vi "Eigenvalues.vi"(1 "Number of Rotations (100)":i32, 2 "n":i32, 3 "A":sgl[](array[numeric])) -> (0 "eigenvalues":sgl[](array[numeric]))   [LabVIEW 2020]
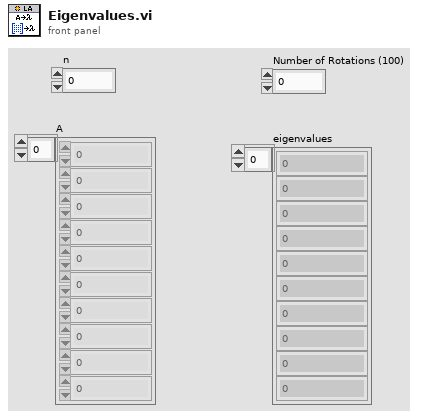
[diagram p1: front panel]
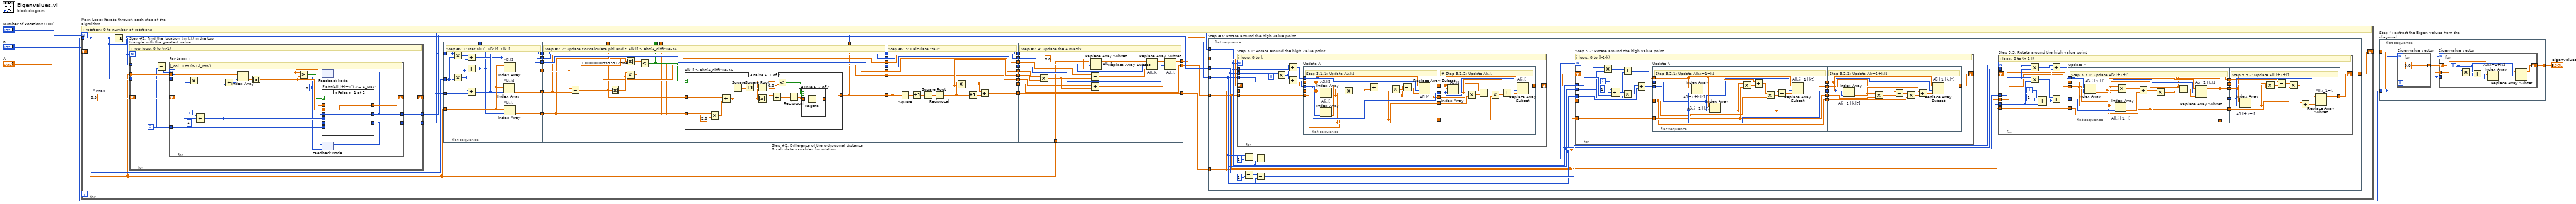
[diagram p0: block diagram]
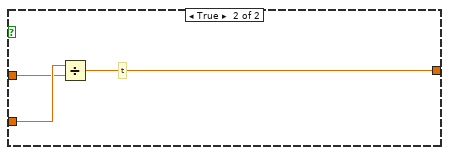
[diagram p3: hidden frame]
diagram:
  n1 = for "Main Loop: Iterate through each step of the algorithm" {
    N: "Number of Rotations (100)" -> [_]
    tunnel: "n" -> [w35]
    shift-right: [w6] -> w2
    shift-left: "A" -> [w25]
    w37 = sgl 0.0  # A max
    # "i_rotation: 0 to number_of_rotations"
    n2 = Decrement(x=w35) -> (x-1=w36:i32)
    n3 = for "Step #1: Find the location (in k,l) in the top triangle with the greatest value" {
      N: w36 -> [_]
      tunnel: w36 -> [w255]
      shift-right: [w259] -> _
      shift-left: w37 -> [w257]
      tunnel: [w258] -> w8
      tunnel: [w256] -> w7
      tunnel: w25 -> [w254]
      tunnel: w35 -> [w253]
      i -> [w252]
      # "i_row loop, 0 to (n-1)"
      n4 = Subtract(x=w255, y=w252) -> (x-y=w260:i32)
      n5 = for "For Loop: j" {
        N: w260 -> [_]
        shift-right: [w269] -> w259
        shift-left: w257 -> [w268]
        tunnel: [w261] -> w258
        tunnel: [w265] -> w256
        tunnel: w254 -> [w278]
        tunnel: w252 -> [w267]
        tunnel: w253 -> [w276]
        i -> [w272]
        w262 = 0
        # "j_col, 0 to (n-1-i_row)"
        n6 = Multiply(x=w276, y=w267) -> (x*y=w274:i32)
        n7 = Compound Arithmetic op=ADD(w272, w267, 1 ("value")) -> (w264:i32)
        n8 = Add(x=w274, y=w264) -> (x+y=w273:i32)
        n9 = Index Array(array=w278, index=w273) -> (element=w275:sgl)
        n10 = Absolute Value(x=w275) -> (abs(x)=w270:sgl)
        n11 = Greater Or Equal?(x=w270, y=w268) -> (x >= y?=w271:bool)
        n12 = feedback #1(w262) -> (w263:i32)
        n13 = feedback #2(w262) -> (w266:i32)
        n14 = case "if abs(A[i,j+i+1]) >= A_Max:" shown="False" w271 {
          tunnel: [w281 w284] -> w269
          tunnel: w270 -> [_ w284]
          tunnel: w268 -> [w281 _]
          tunnel: w267 -> [_ w283]
          tunnel: [w280 w283] -> w265
          tunnel: w266 -> [w280 _]
          tunnel: w264 -> [_ w282]
          tunnel: [w279 w282] -> w261
          tunnel: w263 -> [w279 _]
          frame False {
          }
          frame True {
          }
        }
        n15 = feedback-in #1(w261) -> ()
        n16 = feedback-in #2(w265) -> ()
      }
    }
    n17 = flat-sequence "Step #2: Difference of the orthogonal distance & calculate variables for rotation" {
      tunnel: [w45] -> w32
      tunnel: [w44] -> w31
      tunnel: [w43] -> w30
      tunnel: w7 -> [w49]
      tunnel: w35 -> [w48]
      tunnel: w8 -> [w47]
      tunnel: w25 -> [w46]
      tunnel: [w38] -> w21
      tunnel: [w40] -> w20
      tunnel: [w39] -> w17
      tunnel: [w38] -> _
      tunnel: [w53] -> w29
      tunnel: w32 -> [w55]
      tunnel: w31 -> [w54]
      tunnel: w30 -> [w50]
      tunnel: [w58] -> w22
      tunnel: w21 -> [w58]
      tunnel: w20 -> [w57]
      tunnel: [w57] -> w19
      tunnel: w17 -> [w56]
      tunnel: [w56] -> w16
      tunnel: [w50] -> w14
      tunnel: [w55] -> w12
      tunnel: [w54] -> w10
      tunnel: [w53] -> _
      tunnel: [w52] -> _
      tunnel: [w51] -> _
      tunnel: [w50] -> _
      tunnel: w29 -> [w91]
      tunnel: [w91] -> w28
      tunnel: [w90] -> w27
      tunnel: [w89] -> w26
      tunnel: [w88] -> w23
      tunnel: w22 -> [w88]
      tunnel: w19 -> [w87]
      tunnel: [w87] -> w18
      tunnel: w16 -> [w86]
      tunnel: [w86] -> w15
      tunnel: w14 -> [w85]
      tunnel: [w85] -> w13
      tunnel: w12 -> [w84]
      tunnel: [w84] -> w11
      tunnel: w10 -> [w83]
      tunnel: [w83] -> w9
      tunnel: [w112] -> w33
      tunnel: [w113] -> w34
      tunnel: w28 -> [w111]
      tunnel: w27 -> [w113]
      tunnel: w26 -> [w112]
      tunnel: w25 -> [w99]
      tunnel: [w100] -> w24
      tunnel: w23 -> [w106]
      tunnel: w18 -> [w105]
      tunnel: w15 -> [w104]
      tunnel: w13 -> [w103]
      tunnel: w11 -> [w102]
      tunnel: w9 -> [w101]
      frame #0 {
        # "Step #2.1: Get K[I,I], K[k,k], K[k,l]"
        n18 = Multiply(x=w47, y=w48) -> (x*y=w42:i32)
        n19 = Multiply(x=w49, y=w48) -> (x*y=w41:i32)
        n20 = Add(x=w42, y=w47) -> (x+y=w39:i32)
        n21 = Add(x=w41, y=w47) -> (x+y=w38:i32)
        n22 = Add(x=w41, y=w49) -> (x+y=w40:i32)
        n23 = Index Array "A[k,k]"(array=w46, index=w40) -> (element=w44:sgl)
        n24 = Index Array "A[l,l]"(array=w46, index=w39) -> (element=w45:sgl)
        n25 = Index Array "A[k,l]"(array=w46, index=w38) -> (element=w43:sgl)
      }
      frame #1 {
        # "Step #2.2: update t or calculate phi and t, A[k,l] < abs(A_diff)*1e-36"
        n26 = Subtract(x=w55, y=w54) -> (x-y=w52:sgl)
        n27 = Absolute Value(x=w52) -> (abs(x)=w60:sgl)
        n28 = Absolute Value(x=w50) -> (abs(x)=w62:sgl)
        n29 = Multiply(x=w60, y=sgl 1e-36 ("x")) -> (x*y=w61:sgl)
        n30 = Less?(x=w62, y=w61) -> (x < y?=w51:bool)
        n31 = case "A[k,l] < abs(A_diff)*1e-36" shown="False" w51 {
          tunnel: w50 -> [w76 w82]
          tunnel: w52 -> [w73 w81]
          tunnel: [w63 w80] -> w53
          frame False {
            n32 = Multiply(x=w76, y=sgl 2.0) -> (x*y=w74:sgl)
            n33 = Divide(x=w73, y=w74) -> (x/y=w67:sgl)
            n34 = Square(x=w67) -> (x^2=w71:sgl)
            n35 = Increment(x=w71) -> (x+1=w70:sgl)
            n36 = Square Root(x=w70) -> (sqrt(x)=w69:sgl)
            n37 = Absolute Value(x=w67) -> (abs(x)=w72:sgl)
            n38 = Add(x=w69, y=w72) -> (x+y=w68:sgl)
            n39 = Less?(x=w67, y=sgl 0.0) -> (x < y?=w65:bool)
            n40 = Reciprocal(x=w68) -> (1/x=w64:sgl)
            n41 = case shown="True" w65 {
              tunnel: w64 -> [w77 w79]
              tunnel: [w77 w78] -> w63
              frame False {
              }
              frame True {
                n42 = Negate(x=w79) -> (-x=w78:sgl)
              }
            }
          }
          frame True {
            # "t"
            n43 = Divide(x=w82, y=w81) -> (x/y=w80:sgl)
          }
        }
      }
      frame #2 {
        # "Step #2.3: Calculate \"tau\""
        n44 = Square(x=w91) -> (x^2=w94:sgl)
        n45 = Increment(x=w94) -> (x+1=w93:sgl)
        n46 = Square Root(x=w93) -> (sqrt(x)=w92:sgl)
        n47 = Reciprocal(x=w92) -> (1/x=w96:sgl)
        n48 = Multiply(x=w96, y=w91) -> (x*y=w90:sgl)
        n49 = Increment(x=w96) -> (x+1=w95:sgl)
        n50 = Divide(x=w90, y=w95) -> (x/y=w89:sgl)
      }
      frame #3 {
        # "Step #2.4: update the A matrix"
        n51 = Multiply(x=w103, y=w111) -> (x*y=w110:sgl)
        n52 = Subtract(x=w101, y=w110) -> (x-y=w108:sgl)
        n53 = Add(x=w102, y=w110) -> (x+y=w107:sgl)
        n54 = Replace Array Subset "A[k,l]"(array=w99, new element=sgl 0.0 ("y"), index=w106) -> (w98:sgl[])
        n55 = Replace Array Subset "A[k,k]"(array=w98, new element=w108, index=w105) -> (w97:sgl[])
        n56 = Replace Array Subset "A[l,l]"(array=w97, new element=w107, index=w104) -> (w100:sgl[])
      }
    }
    n57 = flat-sequence "Step #3: Rotate around the high value point" {
      tunnel: w7 -> [w120]
      tunnel: w24 -> [w128]
      tunnel: w35 -> [w121]
      tunnel: w34 -> [w116]
      tunnel: w33 -> [w117]
      tunnel: w8 -> [w119]
      tunnel: [w118] -> w6
      frame #0 {
        n58 = for "Step 3.1: Rotate around the high value point" {
          N: w120 -> [_]
          tunnel: w121 -> [w227]
          tunnel: w120 -> [w226]
          tunnel: w116 -> [w221]
          tunnel: w117 -> [w225]
          tunnel: w119 -> [w222]
          shift-right: [w214] -> w115
          shift-left: w128 -> [w220]
          i -> [w228]
          # "i loop, 0 to k"
          n59 = Multiply(x=w227, y=w228) -> (x*y=w223:i32)
          n60 = Add(x=w223, y=w226) -> (x+y=w219:i32)
          n61 = Add(x=w223, y=w222) -> (x+y=w224:i32)
          n62 = flat-sequence "Update A" {
            tunnel: w225 -> [w232]
            tunnel: w224 -> [w233]
            tunnel: w221 -> [w230]
            tunnel: w220 -> [w236]
            tunnel: w219 -> [w231]
            tunnel: [w234] -> w218
            tunnel: [w233] -> w217
            tunnel: [w232] -> w216
            tunnel: [w230] -> w215
            tunnel: [w229] -> w213
            tunnel: w218 -> [w251]
            tunnel: w217 -> [w243]
            tunnel: w216 -> [w250]
            tunnel: w215 -> [w247]
            tunnel: [w242] -> w214
            tunnel: w213 -> [w241]
            frame #0 {
              # "Step 3.1.1: Update A[i,k]"
              n63 = Index Array "A[i,k]"(array=w236, index=w231) -> (element=w229:sgl)
              n64 = Index Array "A[i,l]"(array=w236, index=w233) -> (element=w239:sgl)
              n65 = Multiply(x=w229, y=w232) -> (x*y=w240:sgl)
              n66 = Add(x=w239, y=w240) -> (x+y=w238:sgl)
              n67 = Multiply(x=w238, y=w230) -> (x*y=w237:sgl)
              n68 = Subtract(x=w229, y=w237) -> (x-y=w235:sgl)
              n69 = Replace Array Subset "A[i,k]"(array=w236, new element=w235, index=w231) -> (w234:sgl[])
            }
            frame #1 {
              # "# Step 3.1.2: Update A[i,l]"
              n70 = Index Array "A[i,l]"(array=w251, index=w243) -> (element=w245:sgl)
              n71 = Multiply(x=w245, y=w250) -> (x*y=w249:sgl)
              n72 = Subtract(x=w241, y=w249) -> (x-y=w248:sgl)
              n73 = Multiply(x=w248, y=w247) -> (x*y=w246:sgl)
              n74 = Add(x=w245, y=w246) -> (x+y=w244:sgl)
              n75 = Replace Array Subset "A[i,l]"(array=w251, new element=w244, index=w243) -> (w242:sgl[])
            }
          }
        }
        n76 = Subtract(x=w119, y=1) -> (x-y=w127:i32)
        n77 = Subtract(x=w121, y=1) -> (x-y=w123:i32)
        n78 = Subtract(x=w127, y=w120) -> (x-y=w125:i32)
        n79 = Subtract(x=w123, y=w119) -> (x-y=w122:i32)
        n80 = for "Step 3.2: Rotate around the high value point" {
          N: w125 -> [_]
          shift-right: [w189] -> w114
          shift-left: w115 -> [w187]
          tunnel: w120 -> [w185]
          tunnel: w121 -> [w181]
          tunnel: w119 -> [w179]
          tunnel: w117 -> [w177]
          tunnel: w116 -> [w175]
          i -> [w184]
          # "i loop, 0 to (l-1-k)"
          n81 = Multiply(x=w185, y=w181) -> (x*y=w183:i32)
          n82 = Compound Arithmetic op=ADD(w184, 1 ("value"), w185) -> (w182:i32)
          n83 = Add(x=w183, y=w182) -> (x+y=w178:i32)
          n84 = Multiply(x=w182, y=w181) -> (x*y=w180:i32)
          n85 = Add(x=w180, y=w179) -> (x+y=w176:i32)
          n86 = flat-sequence "Update A" {
            tunnel: [w201] -> w188
            tunnel: w187 -> [w200]
            tunnel: w178 -> [w192]
            tunnel: w177 -> [w193]
            tunnel: w176 -> [w194]
            tunnel: w175 -> [w191]
            tunnel: [w194] -> w174
            tunnel: [w193] -> w173
            tunnel: [w191] -> w172
            tunnel: [w190] -> w171
            tunnel: [w212] -> w189
            tunnel: w188 -> [w209]
            tunnel: w174 -> [w211]
            tunnel: w173 -> [w210]
            tunnel: w172 -> [w206]
            tunnel: w171 -> [w202]
            frame #0 {
              # "Step 3.2.1: Update A[k,i+1+k]"
              n87 = Index Array "A[i+1+k,l?]"(array=w200, index=w194) -> (element=w199:sgl)
              n88 = Index Array "A[k,i+1+k?]"(array=w200, index=w192) -> (element=w190:sgl)
              n89 = Multiply(x=w190, y=w193) -> (x*y=w198:sgl)
              n90 = Add(x=w199, y=w198) -> (x+y=w197:sgl)
              n91 = Multiply(x=w197, y=w191) -> (x*y=w196:sgl)
              n92 = Subtract(x=w190, y=w196) -> (x-y=w195:sgl)
              n93 = Replace Array Subset "A[k,i+1+k?]"(array=w200, new element=w195, index=w192) -> (w201:sgl[])
            }
            frame #1 {
              # "Step 3.2.2: Update A[i+1+k,l]"
              n94 = Index Array "A[i+1+k,l?]"(array=w209, index=w211) -> (element=w204:sgl)
              n95 = Multiply(x=w204, y=w210) -> (x*y=w208:sgl)
              n96 = Subtract(x=w202, y=w208) -> (x-y=w207:sgl)
              n97 = Multiply(x=w207, y=w206) -> (x*y=w205:sgl)
              n98 = Add(x=w204, y=w205) -> (x+y=w203:sgl)
              n99 = Replace Array Subset "A[i+1+k,l?]"(array=w209, new element=w203, index=w211) -> (w212:sgl[])
            }
          }
        }
        n100 = for "Step 3.3: Rotate around the high value point" {
          N: w122 -> [_]
          tunnel: w121 -> [w143]
          tunnel: w120 -> [w147]
          tunnel: w119 -> [w142]
          shift-right: [w130] -> w118
          shift-left: w114 -> [w138]
          tunnel: w117 -> [w136]
          tunnel: w116 -> [w134]
          i -> [w146]
          # "i loop, 0 to (n-1-l)"
          n101 = Multiply(x=w147, y=w143) -> (x*y=w144:i32)
          n102 = Multiply(x=w143, y=w142) -> (x*y=w141:i32)
          n103 = Compound Arithmetic op=ADD(w146, 1 ("value"), w142) -> (w140:i32)
          n104 = Add(x=w144, y=w140) -> (x+y=w137:i32)
          n105 = Add(x=w141, y=w140) -> (x+y=w135:i32)
          n106 = flat-sequence "Update A" {
            tunnel: [w149] -> w139
            tunnel: w138 -> [w155]
            tunnel: w137 -> [w151]
            tunnel: w136 -> [w152]
            tunnel: w135 -> [w153]
            tunnel: w134 -> [w150]
            tunnel: [w153] -> w133
            tunnel: [w152] -> w132
            tunnel: [w150] -> w131
            tunnel: [w149] -> _
            tunnel: [w148] -> w129
            tunnel: [w170] -> w130
            tunnel: w139 -> [w167]
            tunnel: w133 -> [w169]
            tunnel: w132 -> [w168]
            tunnel: w131 -> [w164]
            tunnel: w129 -> [w160]
            frame #0 {
              # "Step 3.3.1: Update A[k,i+1+l]"
              n107 = Index Array "A[k,i+1+l]"(array=w155, index=w151) -> (element=w148:sgl)
              n108 = Index Array "A[l,i+1+l]"(array=w155, index=w153) -> (element=w158:sgl)
              n109 = Multiply(x=w148, y=w152) -> (x*y=w159:sgl)
              n110 = Add(x=w159, y=w158) -> (x+y=w157:sgl)
              n111 = Multiply(x=w157, y=w150) -> (x*y=w156:sgl)
              n112 = Subtract(x=w148, y=w156) -> (x-y=w154:sgl)
              n113 = Replace Array Subset "A[i+1+k,l]"(array=w155, new element=w154, index=w151) -> (w149:sgl[])
            }
            frame #1 {
              # "Step 3.3.2: Update A[l,i+1+l]"
              n114 = Index Array "A[l,i+1+l]"(array=w167, index=w169) -> (element=w162:sgl)
              n115 = Multiply(x=w162, y=w168) -> (x*y=w166:sgl)
              n116 = Subtract(x=w160, y=w166) -> (x-y=w165:sgl)
              n117 = Multiply(x=w165, y=w164) -> (x*y=w163:sgl)
              n118 = Add(x=w163, y=w162) -> (x+y=w161:sgl)
              n119 = Replace Array Subset "A[l,i_1+l]"(array=w167, new element=w161, index=w169) -> (w170:sgl[])
            }
          }
        }
      }
    }
  }
  n120 = flat-sequence "Step 4: extract the Eigen values from the diagonal" {
    tunnel: w2 -> [w287]
    tunnel: "n" -> [w286]
    tunnel: [w285] -> w4
    frame #0 {
      n121 = for "Eigenvalue vector" {
        N: w286 -> [_]
        tunnel: [sgl 0.0] -> w288 mode=indexing
      }
      n122 = for "Eigenvalue vector" {
        N: w286 -> [_]
        shift-right: [w295] -> w285
        shift-left: w288 -> [w296]
        tunnel: w287 -> [w294]
        tunnel: w286 -> [w293]
        i -> [w291]
        n123 = Multiply(x=w293, y=w291) -> (x*y=w292:i32)
        n124 = Add(x=w292, y=w291) -> (x+y=w290:i32)
        n125 = Index Array "A[k,i+1+l?]"(array=w294, index=w290) -> (element=w289:sgl)
        n126 = Replace Array Subset(array=w296, new element=w289, index=w291) -> (w295:sgl[])
      }
    }
  }
  "eigenvalues" <- w4
